vi "Observer Pattern Demo.vi"() -> ()   [LabVIEW 2011]
uses:
  Class/Text Message/Text Message.lvclass
  Class/Normal Text/Normal Text.lvclass
  Class/Reverse Text/Reverse Text.lvclass
  Class/Observable/Observable.lvclass
panel:
  in  "Next Button":bool
  in  "Text 2":string="abcd"
  in  "Text 1":string="1234"
  out "Reversed  Text Display":string
  out "Normal Text Display":string
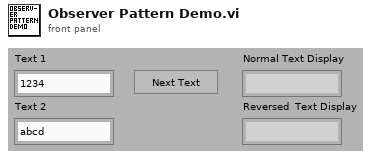
[diagram p1: front panel]
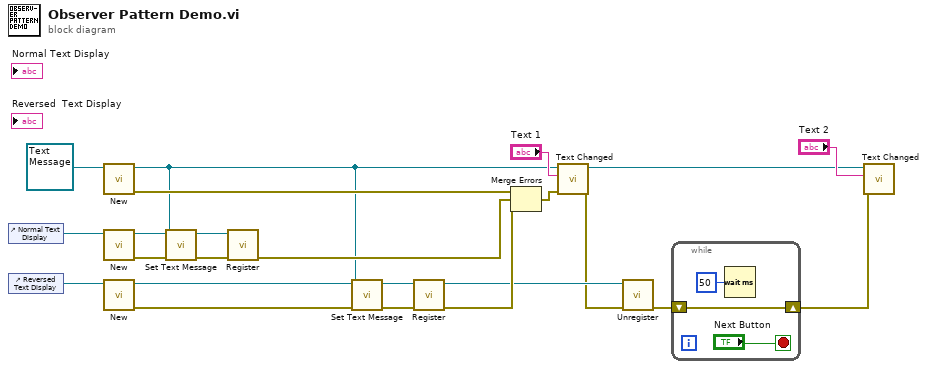
[diagram p0: block diagram]
diagram:
  n1 = control-ref of="Normal Text Display"() -> (w23:refnum<vi>)
  n2 = control-ref of="Reversed  Text Display"() -> (w22:refnum<vi>)
  n3 = call "New.vi"("Observable in"=refnum<class "Text Message.lvclass"> refnum ("Text Message.lvclass")) -> ("error out"=w9:errorcluster, "Observable out"=w7:refnum<class "Text Message.lvclass">)  [unwired: 9 in]
  n4 = call "New.vi"("String Refnum"=w23) -> ("error out"=w18:errorcluster, "Normal Text out"=w19:refnum<class "Normal Text.lvclass">)  [unwired: 9 in]
  n5 = call "New.vi"("String Refnum"=w22) -> ("error out"=w16:errorcluster, "Reverse Text out"=w21:refnum<class "Reverse Text.lvclass">)  [unwired: 9 in]
  n6 = call "Set Text Message.vi"("error in (no error)"=w18, "Observable"=w7, "Normal Text in"=w19) -> ("error out"=w13:errorcluster, "Normal Text out"=w17:refnum<class "Normal Text.lvclass">)  [unwired: 7 in]
  n7 = call-dynamic "Register.vi"("error in (no error)"=w13, "Normal Text in"=w17) -> ("error out"=w10:errorcluster)  [unwired: 8 in, 1 out]
  n8 = call "Set Text Message.vi"("error in (no error)"=w16, "Observable"=w7, "Reverse Text in"=w21) -> ("error out"=w12:errorcluster, "Reverse Text out"=w20:refnum<class "Reverse Text.lvclass">)  [unwired: 7 in]
  n9 = call-dynamic "Register.vi"("error in (no error)"=w12, "Reverse Text in"=w20) -> ("error out"=w11:errorcluster, "Reverse Text out"=w6:refnum<class "Reverse Text.lvclass">)  [unwired: 8 in]
  n10 = Merge Errors(w9, w10, w11) -> (w15:errorcluster)
  n11 = call "Text Changed.vi"("error in (no error)"=w15, "Text"="Text 1", "Text Message in"=w7) -> ("error out"=w5:errorcluster, "Text Message out"=w3:refnum<class "Text Message.lvclass">)  [unwired: 7 in]
  n12 = call-dynamic "Unregister.vi"("error in (no error)"=w5, "Reverse Text in"=w6) -> ("error out"=w2:errorcluster)  [unwired: 8 in, 1 out]
  n13 = while {
    shift-right: [w26] -> w1
    shift-left: w2 -> [w26]
    stop <- "Next Button" stop-if-true
    n14 = Wait (ms)(milliseconds to wait=u32 50) -> ()  [unwired: 1 out]
  }
  n15 = call "Text Changed.vi"("error in (no error)"=w1, "Text"="Text 2", "Text Message in"=w3) -> ()  [unwired: 7 in, 2 out]
